vi "add_file.vi"(8 "error in":errorcluster, 9 "file_path":path, 10 "name":string, 11 "MultipartForm in":refnum<class "MultipartForm.lvclass">) -> (0 "error out":errorcluster, 3 "MultipartForm out":refnum<class "MultipartForm.lvclass">)   [LabVIEW 2020, in "reqwest.lvlib" / "MultipartForm.lvclass"]
uses:
  MultipartForm.lvclass
  MultipartForm.lvclass/MultipartForm.ctl
  reqwest.lvlib
  lv_reqwest_64.dll
panel:
  out "success":bool
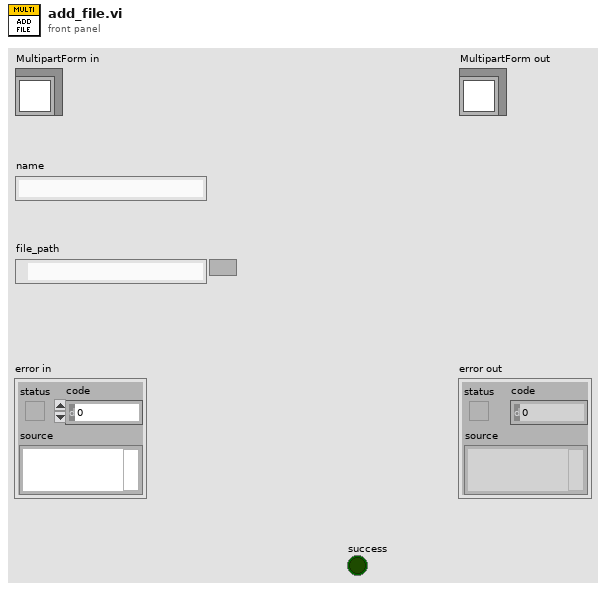
[diagram p1: front panel]
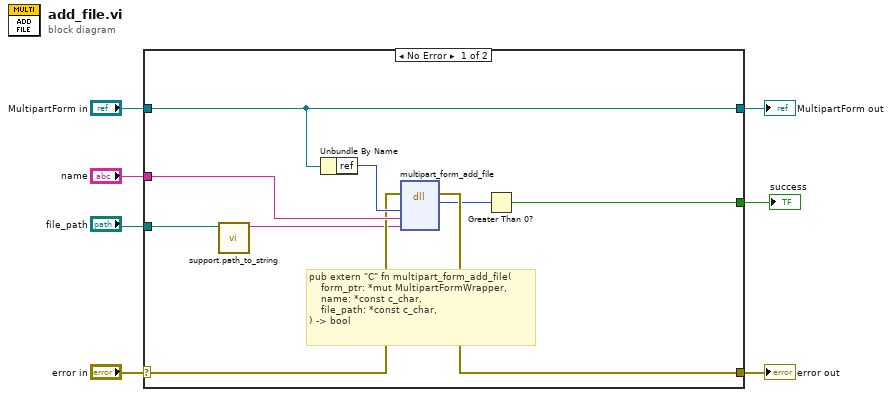
[diagram p0: block diagram]
diagram:
  n1 = case shown="No Error" "error in" {
    selector: "error in" -> [w13 w18]
    tunnel: [w12 w18] -> w6
    tunnel: [w16 w17] -> w4
    tunnel: "MultipartForm in" -> [w16 w17]
    tunnel: "name" -> [w14 _]
    tunnel: "file_path" -> [w9 _]
    tunnel: [w10 _] -> w1
    frame No Error {
      # "pub extern \"C\" fn multipart_form_add_file(\n    form_ptr: *mut MultipartFormWrapper,\n    name: *const c_char,\n    file_path: *const c_char,\n) -> bool"
      n2 = call "support.path_to_string.vi"("path"=w9) -> ("path as string"=w8:string)  [unwired: 10 in]
      n3 = Unbundle By Name(w16) -> ("ref"=w15:u64)
      n4 = dll-call lib="C:/Projects/reqwest-rs-labview/lv_src/lv_reqwest_*.*" fn="multipart_form_add_file"(error in=w13, "form_ptr"=w15, "name"=w14, "file_path"=w8) -> (error out=w12:errorcluster, "bool"=w11:u8)  [unwired: 5 in, 1 out]
      n5 = Greater Than 0?(x=w11) -> (x > 0?=w10:bool)
    }
    frame Error {
    }
  }
  "error out" <- w6
  "MultipartForm out" <- w4
  "success" <- w1
